vi "Stop Variable.vi"(7 "action":T1, 9 "error in (no error)":errorcluster) -> (1 "error out":errorcluster, 2 "stop":bool)   [LabVIEW 2022 SP3]
uses:
  Stop Variable Action.ctl
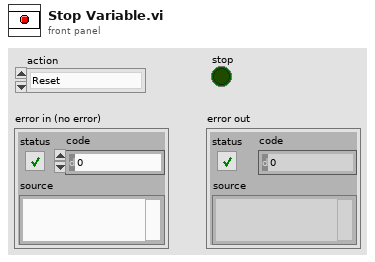
[diagram p1: front panel]
types:
  T1 = typedef "Stop Variable Action.ctl" = enum16{"Reset", "Check", "Stop"}
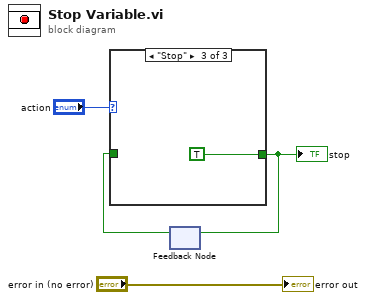
[diagram p0: block diagram]
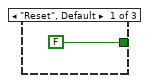
[diagram p2: hidden frame]
diagram:
  n1 = feedback #1() -> (w2:bool)  [unwired: 1 in]
  n2 = case shown="\"Stop\"" "action" {
    tunnel: [FALSE w6 TRUE] -> w3
    tunnel: w2 -> [_ w6 _]
    frame "Reset", Default {
    }
    frame "Check" {
    }
    frame "Stop" {
    }
  }
  "stop" <- w3
  n3 = feedback-in #1(w3) -> ()
  "error out" <- "error in (no error)"
